vi "Copy Target Structure To Instance.vi"(8 "tsRef":refnum<vi>, 11 "instVI diagram":refnum<vi>) -> (0 "copied tsRef":refnum<vi>, 3 "instVI diagram out":refnum<vi>)   [LabVIEW 2020, in "NI_TargetHelper.lvlib"]
uses:
  <vilib>/TargetSupport/NI_TargetHelper/NI_TargetHelper.lvlib
  <vilib>/Utility/miscctls.llb/LVPositionTypeDef.ctl
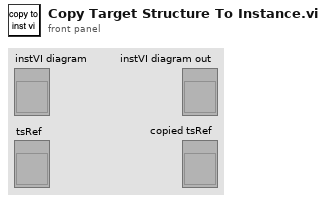
[diagram p1: front panel]
types:
  T1 = typedef "LVPositionTypeDef.ctl" = cluster{"Left":i32, "Top":i32}
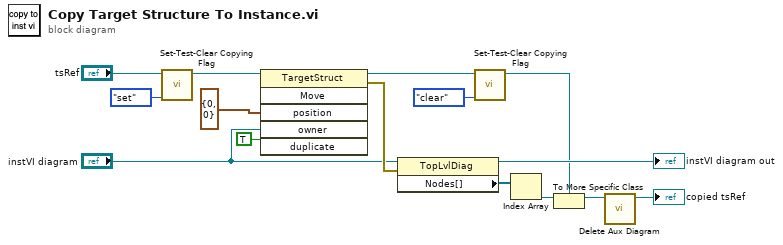
[diagram p0: block diagram]
diagram:
  n1 = call <vilib>:"Set-Test-Clear Copying Flag.vi"("op"=enum16{"test", "clear", "set"}."set", "tsRef"="tsRef") -> ("tsRef out"=w4:refnum<vi>)  [unwired: 8 in, 1 out]
  n2 = invoke class="TargetStruct" method="Move"(reference=w4, "position"=T1 {"Left"=0, "Top"=0}, "owner"="instVI diagram", "duplicate"=TRUE ("Duplicate? (F)")) -> (reference out=w2:refnum<vi>, error out=w12:errorcluster)  [unwired: 2 in, 4 out]
  n3 = property class="TopLvlDiag"(reference="instVI diagram", error in=w12) -> (reference out=→"instVI diagram out":refnum<vi>, "Nodes[]"=w15:refnum<vi>[])  [unwired: 1 out]
  n4 = call <vilib>:"Set-Test-Clear Copying Flag.vi"("op"=enum16{"test", "clear", "set"}."clear", "tsRef"=w2) -> ("tsRef out"=w1:refnum<vi>)  [unwired: 8 in, 1 out]
  n5 = Index Array(array=w15) -> (element=w14:refnum<vi>)  [unwired: 1 in]
  n6 = To More Specific Class(target class=w1, reference=w14) -> (specific class reference=w8:refnum<vi>)  [unwired: 1 in, 1 out]
  n7 = call <vilib>:"Delete Aux Diagram.vi"("tsRef"=w8) -> ("tsRef out"=→"copied tsRef":refnum<vi>)  [unwired: 10 in]
